vi "LJ-T7DAQ.vi"() -> (0 "error out":errorcluster)   [LabVIEW 2017]
uses:
  PWA/PWAtasksGLOBAL.vi
  Globals/Meas_global.vi
  ADAM Serial/Instrument drivers/LabJack/T7/Stream/T7 Stream Globals KAG.vi
  ADAM Serial/Instrument drivers/LabJack/T7/Stream/T7 IP Config KAG.ctl
  ADAM Serial/Instrument drivers/LabJack/T7/Stream/T7 Stream Config KAG.ctl
panel:
  out "Current Block No":i32
  out "Strm Config Out":T1={"Scan Rate (Hz)"=1000.0, "Samples Per Packet"=512, "Resolution Index"=0, "Buffer Size (bytes)"=32768, "NumScans"=1500, "Read Timeout (ms)"=5000, "Scan Table"=[{"Channel"=0, "BipGain"=0, "Input Config"="Single-Ended"}, {"Channel"=1, "BipGain"=0, "Input Config"="Single-Ended"}, {"Channel"=2, "BipGain"=0, "Input Config"="Single-Ended"}, {"Channel"=3, "BipGain"=0, "Input Config"="Single-Ended"}]} {"Samples Per Packet" max=512 step=1; "Buffer Size (bytes)" max=32768 step=1; "Resolution Index" max=8 step=1; "Scan Rate (Hz)" max=100000; "Scan Table"."BipGain" items=["x1", "x10", "x100", "x1000"]; "Scan Table"."Channel" step=1}
  out "IP Configuration":T2={"Connection ID In"=refnum, "Connection ID Out"=refnum, "Device IP"="", "Port"=502}
  out "Requested # Blks":i32
  in  "milliseconds holdup":u32
  out "Waveform Graph":dbl[][](graph)
  out "AuditTrail":string[](array[string])
  out "input terminal configuration":i32(ring)=10106 items=["default"=-1, "RSE"=10083, "NRSE"=10078, "Differential"=10106, "Pseudodifferential"=12529]
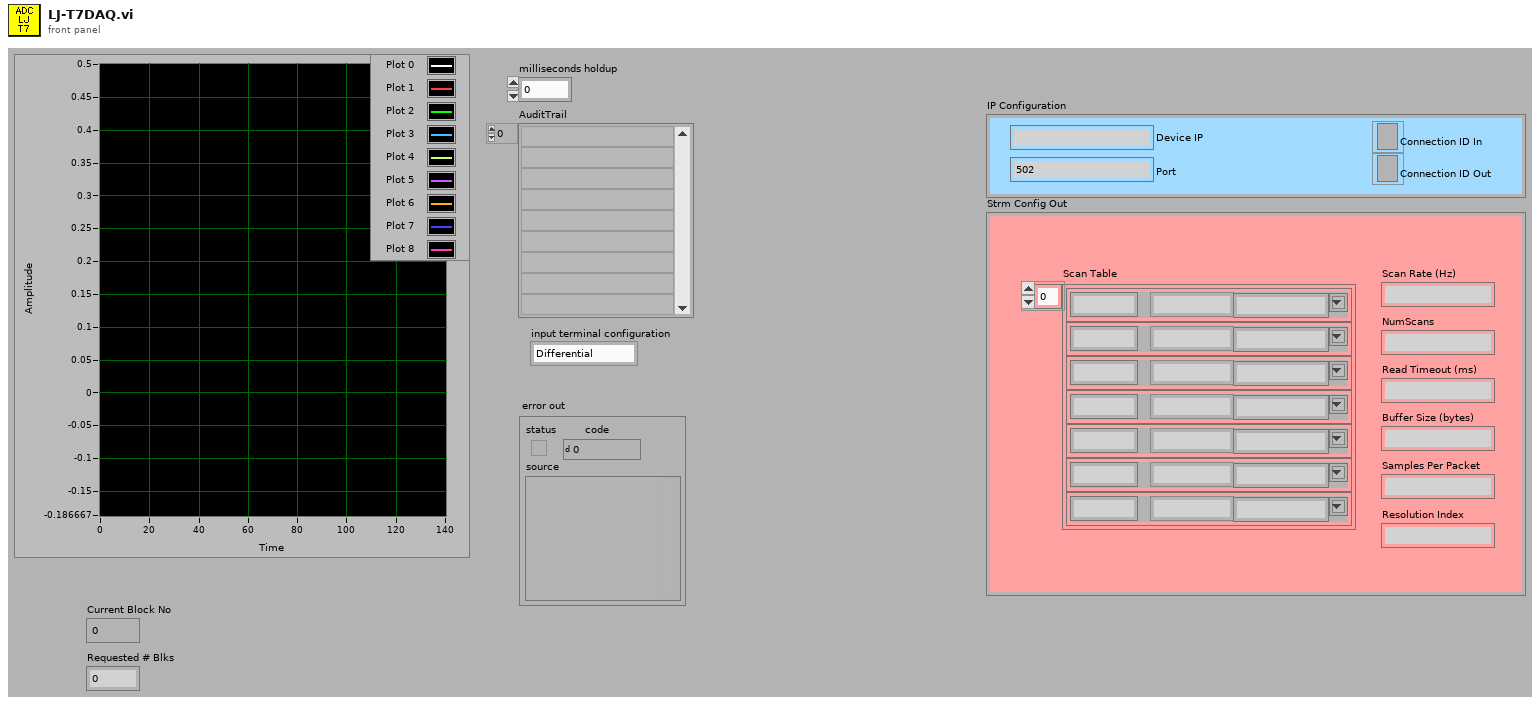
[diagram p1: front panel]
types:
  T1 = typedef "T7 Stream Config KAG.ctl" = cluster{"Scan Rate (Hz)":sgl, "Samples Per Packet":u32, "Resolution Index":u32, "Buffer Size (bytes)":u32, "NumScans":u32, "Read Timeout (ms)":u32, "Scan Table":cluster{"Channel":u32, "BipGain":u32, "Input Config":string}[]}
  T2 = cluster{"Connection ID In":refnum<k5>, "Connection ID Out":refnum<k5>, "Device IP":string, "Port":i32}
  T3 = typedef "Ch_and_Spans.ctl" = cluster{"Sync Delay (ms)":dbl, "Ch No":i16, "Var name":string, "Use Latest Calib":bool}
  T4 = typedef "T7 IP Config KAG.ctl" = cluster{"Connection ID In":refnum<k5>, "Connection ID Out":refnum<k5>, "Device IP":string, "Port":i32}
  T5 = cluster{"PSlope":dbl, "NSlope":dbl, "AvgSlope":dbl, "Center":dbl, "Offset":dbl}[]
  T6 = cluster{"Channel":u32, "BipGain":u32, "Input Config":string}[]
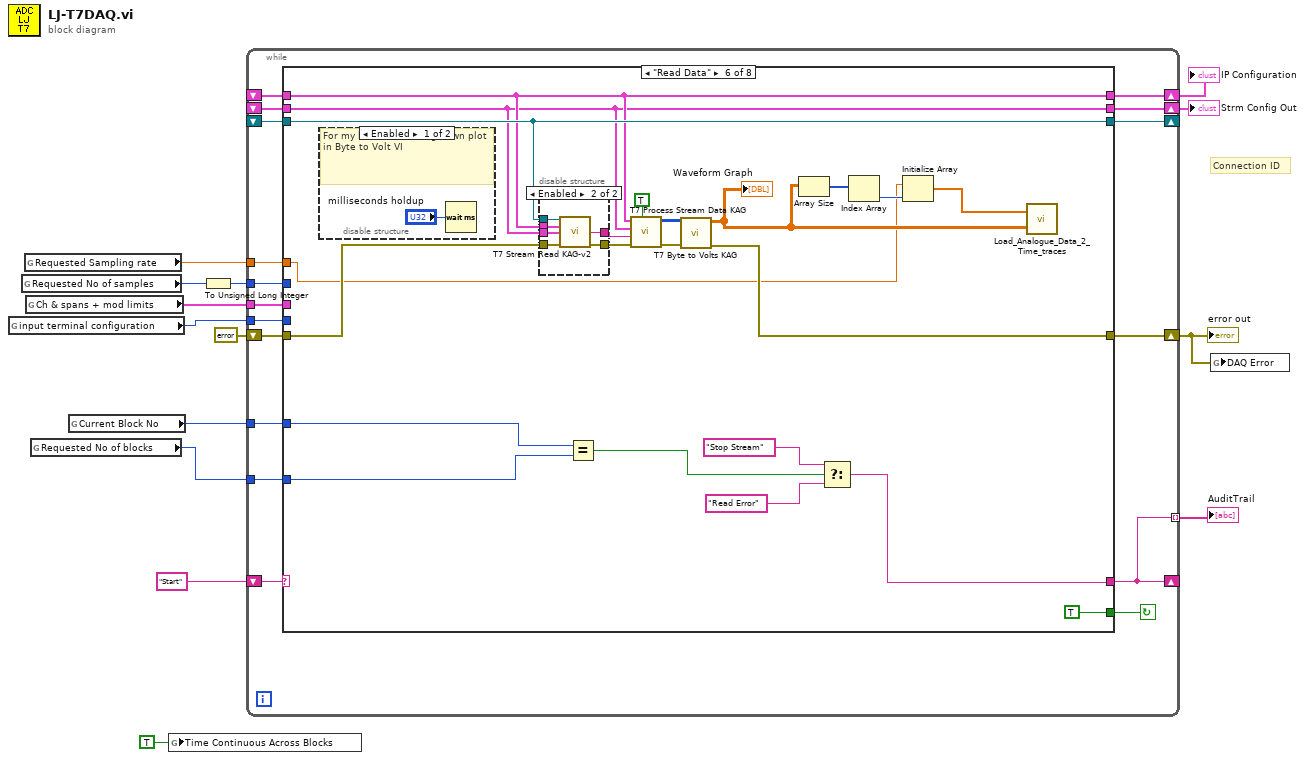
[diagram p0: block diagram]
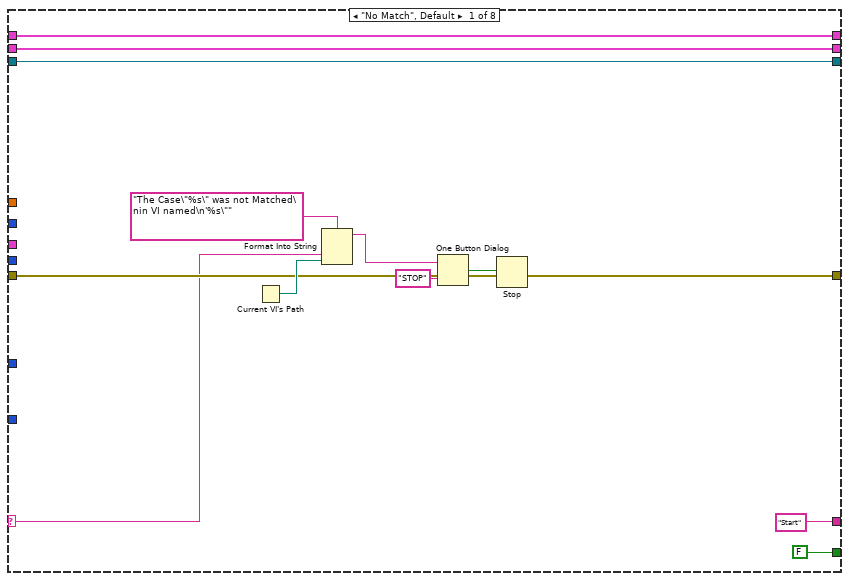
[diagram p2: hidden frame]
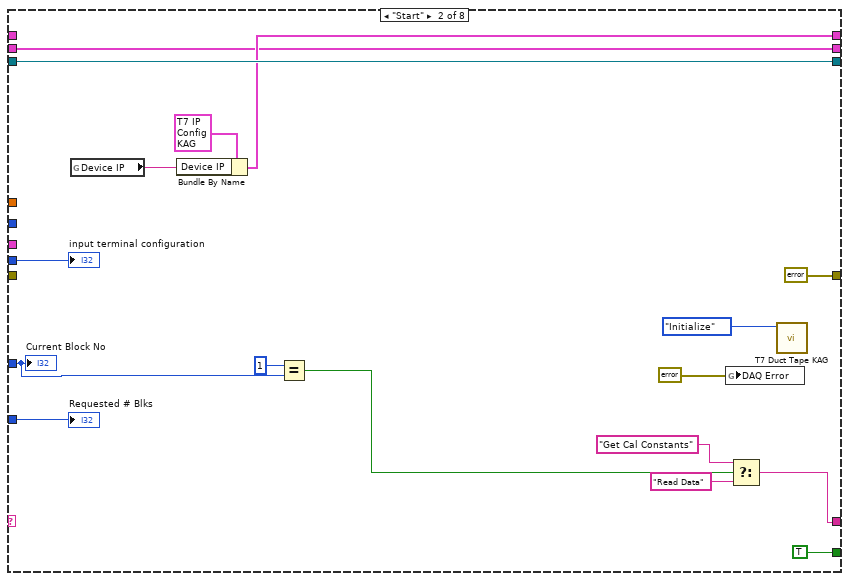
[diagram p3: hidden frame]
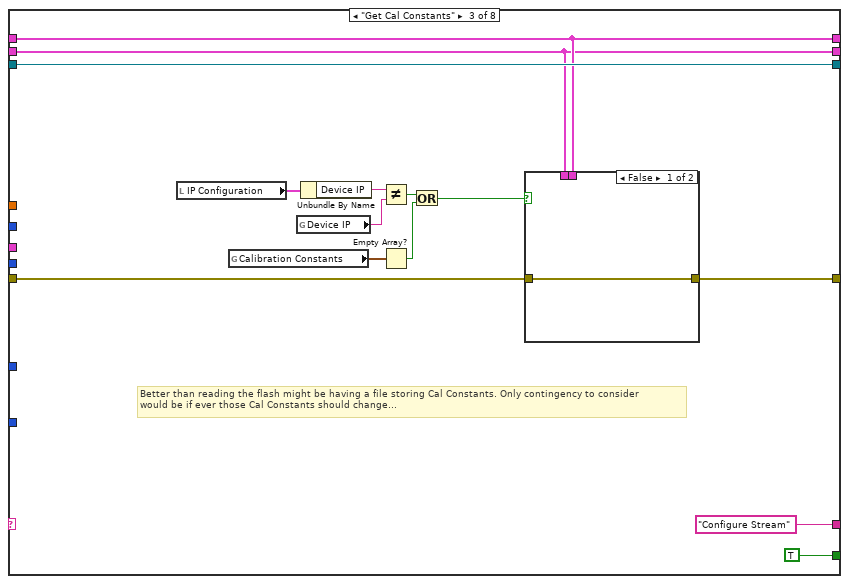
[diagram p4: hidden frame]
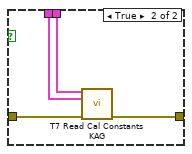
[diagram p5: hidden frame]
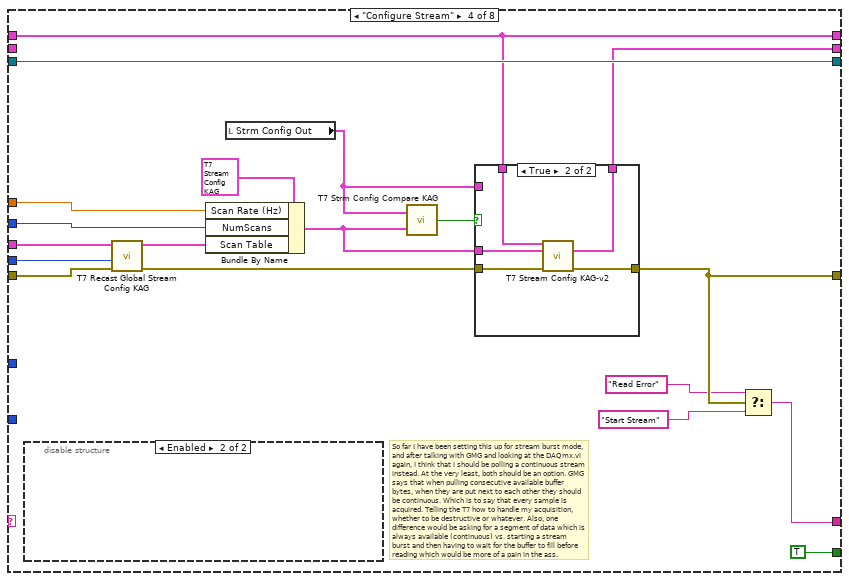
[diagram p6: hidden frame]
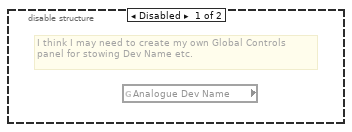
[diagram p8: hidden frame]
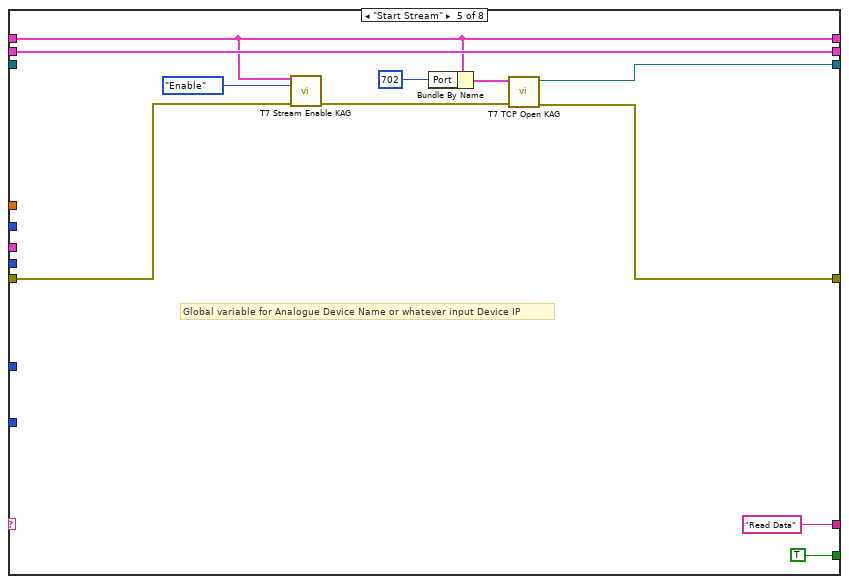
[diagram p9: hidden frame]
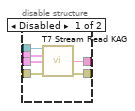
[diagram p10: hidden frame]
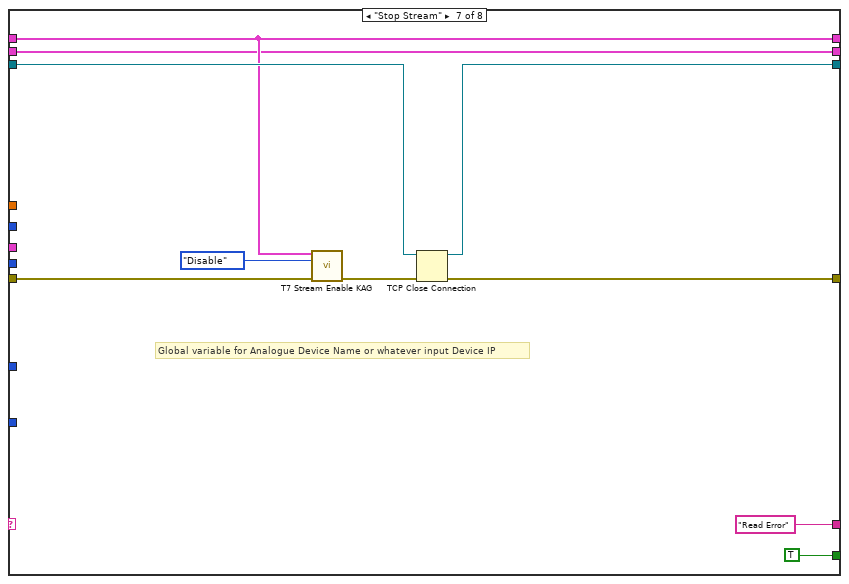
[diagram p12: hidden frame]
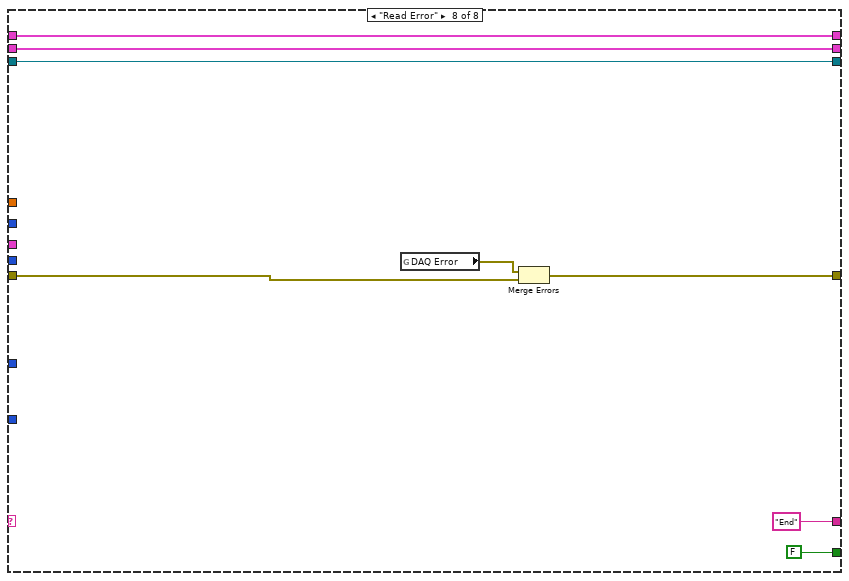
[diagram p13: hidden frame]
diagram:
  # "Connection ID"
  n1 = global read "Meas_global.vi" "input terminal configuration"() -> (w6:i32)
  n2 = global read "Meas_global.vi" "Requested No of samples"() -> (w11:i32)
  n3 = global read "Meas_global.vi" "Requested Sampling rate"() -> (w10:dbl)
  n4 = global read "Meas_global.vi" "Ch & spans + mod limits"() -> (w13:T3[])
  n5 = global read "Meas_global.vi" "Requested No of blocks"() -> (w3:i32)
  n6 = global read "Meas_global.vi" "Current Block No"() -> (w4:i32)
  n7 = global write "Meas_global.vi" "Time Continuous Across Blocks"(TRUE ("Time Continuous Across Blocks")) -> ()
  n8 = To Unsigned Long Integer(number=w11) -> (unsigned 32bit integer=w9:u32)
  n9 = while {
    shift-left: "Start" -> [w30]
    shift-right: [w23] -> _
    shift-right: [w24] -> w12
    shift-left: errorcluster {"status"=FALSE, "code"=0, "source"=""} ("error IO") -> [w29]
    tunnel: w10 -> [w28]
    tunnel: w9 -> [w27]
    tunnel: w13 -> [w25]
    tunnel: [w23] -> w8 mode=indexing
    shift-right: [w22] -> _
    shift-left: _ -> [w21]
    shift-right: [w20] -> w2
    shift-left: _ -> [w19]
    shift-right: [w18] -> w1
    shift-left: _ -> [w17]
    tunnel: w6 -> [w16]
    tunnel: w3 -> [w15]
    tunnel: w4 -> [w26]
    stop <- w31 continue-if-true
    n10 = case shown="\"Read Data\"" w30 {
      selector: w30 -> [w35 _ _ _ _ _ _ _]
      tunnel: [FALSE TRUE TRUE TRUE TRUE TRUE TRUE FALSE] -> w31
      tunnel: ["Start" w44 "Configure Stream" ("f") w89 "Read Data" w132 "Read Error" "End" ("f")] -> w23
      tunnel: [w36 errorcluster {"status"=FALSE, "code"=0, "source"=""} ("error out") w73 w92 w112 w134 w155 w167] -> w24
      tunnel: w29 -> [w36 _ w74 w97 w114 w133 w159 w168]
      tunnel: w28 -> [_ _ _ w86 _ w117 _ _]
      tunnel: w27 -> [_ _ _ w85 _ _ _ _]
      tunnel: w26 -> [_ w49 _ _ _ w124 _ _]
      tunnel: w25 -> [_ _ _ w88 _ _ _ _]
      tunnel: [w34 w57 w70 w95 w111 w130 w157 w164] -> w22
      tunnel: w21 -> [w34 w57 w70 w95 _ w130 w158 w164]
      tunnel: [w33 w54 w69 w94 w107 w129 w154 w163] -> w20
      tunnel: w19 -> [w33 _ w69 w94 w107 w129 w154 w163]
      tunnel: [w32 w53 w68 w87 w108 w128 w153 w162] -> w18
      tunnel: w17 -> [w32 w53 w68 _ w108 w128 w153 w162]
      tunnel: w16 -> [_ w52 _ w93 _ _ _ _]
      tunnel: w15 -> [_ w51 _ _ _ w123 _ _]
      frame "No Match", Default {
        n11 = Current VI's Path() -> (path=w38:path)
        n12 = Format Into String(format string="The Case\"%s\" was not Matched\nin VI named\n'%s\"" ("Format String"), w35, w38) -> (resulting string=w41:string)  [unwired: 2 in, 1 out]
        n13 = One Button Dialog(message=w41, button name ("OK")="STOP") -> (true=w39:bool)
        n14 = Stop(stop? (T)=w39) -> ()
      }
      frame "Start" {
        n15 = global read "T7 Stream Globals KAG.vi" "Device IP"() -> (w56:string)
        n16 = Bundle By Name(cluster=T4 {"Connection ID In"=refnum, "Connection ID Out"=refnum, "Device IP"="192.168.126.147", "Port"=502} ("IP Configuration"), "Device IP"=w56) -> (w54:T4)
        n17 = Equal?(x=1, y=w49) -> (x = y?=w46:bool)
        n18 = global write "Meas_global.vi" "DAQ Error"(errorcluster {"status"=FALSE, "code"=0, "source"=""} ("DAQ Error")) -> ()
        n19 = Select(t="Get Cal Constants", s=w46, f="Read Data") -> (s? t:f=w44:string)
        n20 = call "T7 Duct Tape KAG.vi"("Action"=enum16{"Initialize", "Read", "Update"}."Initialize") -> ()  [unwired: 8 in, 1 out]
        "input terminal configuration" <- w52
        "Requested # Blks" <- w51
        "Current Block No" <- w49
      }
      frame "Get Cal Constants" {
        # "Better than reading the flash might be having a file storing Cal Constants. Only contingency to consider\nwould be if ever those Cal Constants should change..."
        n21 = local read "IP Configuration"() -> (w66:T2)
        n22 = global read "T7 Stream Globals KAG.vi" "Calibration Constants"() -> (w67:T5)
        n23 = global read "T7 Stream Globals KAG.vi" "Device IP"() -> (w64:string)
        n24 = Unbundle By Name(w66) -> ("Device IP"=w65:string)
        n25 = Not Equal?(x=w65, y=w64) -> (x != y?=w63:bool)
        n26 = Empty Array?(array=w67) -> (empty?=w62:bool)
        n27 = Or(x=w63, y=w62) -> (x .or. y?=w61:bool)
        n28 = case shown="False" w61 {
          tunnel: w74 -> [w75 w79]
          tunnel: [w75 w78] -> w73
          tunnel: w69 -> [_ w77]
          tunnel: w68 -> [_ w76]
          frame False {
          }
          frame True {
            n29 = call "T7 Read Cal Constants KAG.vi"("IP Configuration"=w77, "Stream Configuration"=w76, "error in"=w79) -> ("error out"=w78:errorcluster)  [unwired: 11 in, 1 out]
          }
        }
      }
      frame "Configure Stream" {
        # "So far I have been setting this up for stream burst mode, and after talking with GMG and looking at the DAQmx.vi again, I think that I should be polling a continuous stream instead. At the very least, both should be an option. GMG says that when pulling consecutive available buffer bytes, when they are put next to each other they should be continuous. Which is to say that every sample is acquired. Telling the T7 how to handle my acquisition, whether to be destructive or whatever. Also, one difference would be asking for a segment of data which is always available (continuous) vs. starting a stream burst and then having to wait for the buffer to fill before reading which would be more of a pain in the ass."
        n30 = disable-structure shown="Enabled" {
          frame Disabled {
            # "I think I may need to create my own Global Controls panel for stowing Dev Name etc."
            n31 = global read "PWAtasksGLOBAL.vi" "Analogue Dev Name"() -> ()  [unwired: 1 out]
          }
          frame Enabled {
          }
        }
        n32 = call "T7 Recast Global Stream Config KAG.vi"("error in"=w97, "input terminal configuration"=w93, "Ch & spans + mod limits"=w88) -> ("error out"=w96:errorcluster, "Scan Table"=w84:T6)  [unwired: 3 in]
        n33 = Bundle By Name(cluster=T1 {"Scan Rate (Hz)"=1000.0, "Samples Per Packet"=512, "Resolution Index"=0, "Buffer Size (bytes)"=32768, "NumScans"=1500, "Read Timeout (ms)"=5000, "Scan Table"=[{"Channel"=0, "BipGain"=0, "Input Config"="Single-Ended"}, {"Channel"=1, "BipGain"=0, "Input Config"="Single-Ended"}, {"Channel"=2, "BipGain"=0, "Input Config"="Single-Ended"}, {"Channel"=3, "BipGain"=0, "Input Config"="Single-Ended"}]} ("Stream Configuration"), "Scan Rate (Hz)"=w86, "NumScans"=w85, "Scan Table"=w84) -> (w81:T1)
        n34 = local read "Strm Config Out"() -> (w80:T1)
        n35 = call "T7 Strm Config Compare KAG.vi"("Strm Config 1"=w81, "Strm Config 2"=w80) -> ("result"=w82:bool)
        n36 = case shown="True" w82 {
          tunnel: w96 -> [w100 w105]
          tunnel: w94 -> [_ w104]
          tunnel: [w100 w103] -> w92
          tunnel: [w99 w102] -> w87
          tunnel: w81 -> [_ w101]
          tunnel: w80 -> [w99 _]
          frame False {
          }
          frame True {
            n37 = call "T7 Stream Config KAG-v2.vi"("IP Configuration"=w104, "Stream Configuration"=w101, "error in"=w105) -> ("Strm Config Out"=w102:T1, "error out"=w103:errorcluster)  [unwired: 11 in]
          }
        }
        n38 = Select(t="Read Error", s=w92, f="Start Stream") -> (s? t:f=w89:string)
      }
      frame "Start Stream" {
        # "Global variable for Analogue Device Name or whatever input Device IP"
        n39 = call "T7 Stream Enable KAG.vi"("IP Configuration"=w107, "Enable"=enum32{"Disable", "Enable"}."Enable", "error in"=w114) -> ("error out"=w113:errorcluster)  [unwired: 12 in]
        n40 = Bundle By Name(cluster=w107, "Port"=702) -> (w109:T4)
        n41 = call "T7 TCP Open KAG.vi"("error in"=w113, "IP Configuration"=w109) -> ("error out"=w112:errorcluster, "connection ID out"=w111:refnum<k5>)  [unwired: 8 in]
      }
      frame "Read Data" {
        n42 = disable-structure shown="Enabled" {
          frame Enabled {
            # "For my benefit...slowing down plot in Byte to Volt VI"
            n43 = Wait (ms)(milliseconds to wait="milliseconds holdup") -> ()  [unwired: 1 out]
          }
          frame Disabled {
          }
        }
        n44 = disable-structure shown="Enabled" {
          disable-tunnel: [w144 w150] -> w137
          disable-tunnel: w133 -> [w143 w149]
          disable-tunnel: [w142 w148] -> w131
          disable-tunnel: w130 -> [w141 w147]
          disable-tunnel: w129 -> [w140 w146]
          disable-tunnel: w128 -> [w139 w145]
          frame Disabled {
            n45 = call "T7 Stream Read KAG.vi"("Connection ID In"=w141, "IP Configuration"=w140, "Stream Configuration"=w139, "error in"=w143) -> ("TCP Data"=w142:string, "error out"=w144:errorcluster)  [unwired: 9 in, 1 out]
          }
          frame Enabled {
            n46 = call "T7 Stream Read KAG-v2.vi"("Connection ID In"=w147, "IP Configuration"=w146, "Stream Configuration"=w145, "error in"=w149) -> ("TCP Data"=w148:string, "error out"=w150:errorcluster)  [unwired: 9 in, 1 out]
          }
        }
        n47 = Equal?(x=w124, y=w123) -> (x = y?=w122:bool)
        n48 = call "T7 Process Stream Data KAG.vi"("Backlog"=TRUE, "error in"=w137, "TCP Data In"=w131, "Stream Configuration"=w128, "IP Configuration"=w129) -> ("error out"=w136:errorcluster, "Data"=w135:u16[][])  [unwired: 3 in, 2 out]
        n49 = call "T7 Byte to Volts KAG.vi"("error in"=w136, "Byte Data"=w135) -> ("error out"=w134:errorcluster, "Float Data"=w121:dbl[][])  [unwired: 8 in]
        "Waveform Graph" <- w121
        n50 = Array Size(array=w121) -> (size(s)=w120:i32[])
        n51 = Select(t="Stop Stream" ("f"), s=w122, f="Read Error") -> (s? t:f=w132:string)
        n52 = Index Array(array=w120) -> (element=w119:i32)  [unwired: 1 in]
        n53 = Initialize Array(w117, w119) -> (w118:dbl[])
        n54 = call "Load_Analogue_Data_2_Time_traces.vi"("Voltage Array"=w121, "Sampling Rate (Hz)"=w118) -> ()  [unwired: 1 in]
      }
      frame "Stop Stream" {
        # "Global variable for Analogue Device Name or whatever input Device IP"
        n55 = call "T7 Stream Enable KAG.vi"("IP Configuration"=w154, "Enable"=enum32{"Disable", "Enable"}."Disable", "error in"=w159) -> ("error out"=w156:errorcluster)  [unwired: 12 in]
        n56 = TCP Close Connection(connection ID=w158, error in (no error)=w156) -> (connection ID out=w157:refnum<k5>, error out=w155:errorcluster)  [unwired: 1 in]
      }
      frame "Read Error" {
        n57 = global read "Meas_global.vi" "DAQ Error"() -> (w169:errorcluster)
        n58 = Merge Errors(w169, w168) -> (w167:errorcluster)
      }
    }
  }
  "error out" <- w12
  "AuditTrail" <- w8
  "IP Configuration" <- w2
  "Strm Config Out" <- w1
  n59 = global write "Meas_global.vi" "DAQ Error"(w12) -> ()
